vi "Initialize.vi"(8 "error in (no error)":errorcluster, 9 "ID Query":bool, 10 "Reset":bool, 11 "Generic Digital Multi Meter in":refnum<class "Generic Digital Multi Meter.lvclass">) -> (0 "error out":errorcluster, 2 "VISA resource name":refnum<visa-resource-name>, 3 "Generic Digital Multi Meter out":refnum<class "Generic Digital Multi Meter.lvclass">)   [LabVIEW 2014, in "Generic Digital Multi Meter.lvlib" / "Generic Digital Multi Meter.lvclass"]
uses:
  Generic Digital Multi Meter.lvclass
  Abstract Sensor/Abstract Sensor.lvclass
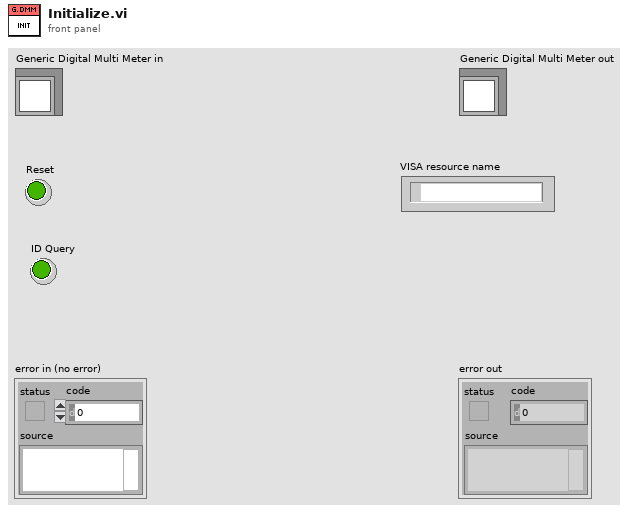
[diagram p1: front panel]
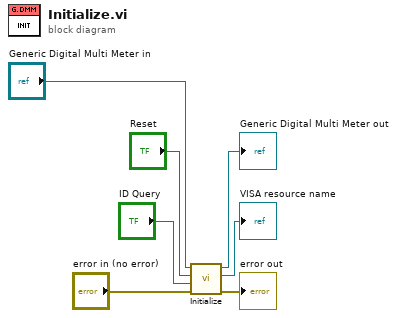
[diagram p0: block diagram]
diagram:
  n1 = call-parent "Initialize.vi"("error in (no error)"="error in (no error)", "ID Query"="ID Query", "Reset"="Reset", "Abstract Sensor in"="Generic Digital Multi Meter in") -> ("error out"=→"error out":errorcluster, "VISA resource name"=→"VISA resource name":refnum<visa-resource-name>, "Abstract Sensor out"=→"Generic Digital Multi Meter out":refnum<class "Generic Digital Multi Meter.lvclass">)  [unwired: 5 in]
